vi "ErrHandler.vi"(1 "Err Code":u32=1, 2 "Action":enum16{"Init", "Process"}(ring)) -> (0 "Err Msg":string="OK!")   [LabVIEW 2011]
uses:
  Globals/CTCGlbs.vi
  Globals/DynaGlbs.vi
panel:
  in  "Incident #":i32=10
  in  "Lookup table":u32[](array[numeric])=[0, 1, 158, 159, 160, 165, 166, 167, 168, 169, 170, 178, 179, 180, 181, 182, 183, 184, 185, 186, 194, 195, 196, 205, 206, 215, 216, 235, 236, 246, 255]
  in  "Text messages":string="Failure\nOK!\nPort in use\nPort not found\nUnknown error\nIllegal stop bits\nIllegal word length\nIllegal parity setting\nIllegal baud rate\nWarning...\nSerial timeout\nNetwork in use\nBad network port\nEnd of file\nBad position\nBad object length\nBad object record\nFile not object\nFile wrong arch\nObject file not found\nRemote access error\nUnknown remote node\nUnsupported remote operation\nNot CT protocol\nBad response\nBad checksum\nOut of CT range\nNetwork not ready\nNetwork timeout\nWindows timer error\nUnknown network error"
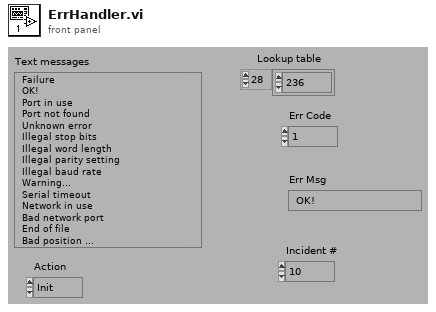
[diagram p1: front panel]
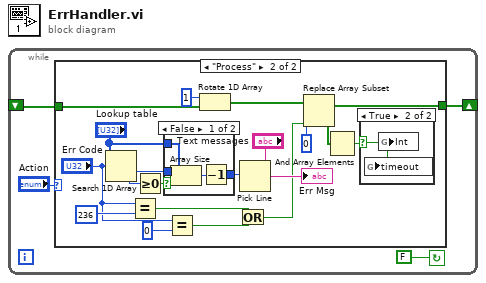
[diagram p0: block diagram]
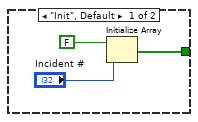
[diagram p2: hidden frame]
diagram:
  n1 = while {
    shift-left: _ -> [w2]
    shift-right: [w3] -> _
    stop <- FALSE continue-if-true
    n2 = case shown="\"Process\"" "Action" {
      tunnel: [w5 w18] -> w3
      tunnel: w2 -> [_ w20]
      frame "Init", Default {
        n3 = Initialize Array(FALSE, "Incident #") -> (w5:bool[])
      }
      frame "Process" {
        n4 = Search 1D Array(1D array="Lookup table", element="Err Code") -> (index of element=w24:i32)  [unwired: 1 in]
        n5 = Equal?(x="Err Code", y=u16 236) -> (x = y?=w10:bool)
        n6 = Greater Or Equal To 0?(x=w24) -> (x >= 0?=w25:bool)
        n7 = case shown="False" w25 {
          tunnel: w24 -> [_ w30]
          tunnel: [w27 w30] -> w13
          tunnel: "Lookup table" -> [w29 _]
          frame False {
            n8 = Array Size(array=w29) -> (size(s)=w28:i32)
            n9 = Decrement(x=w28) -> (x-1=w27:i32)
          }
          frame True {
          }
        }
        n10 = Equal?(x="Err Code", y=u16 0) -> (x = y?=w9:bool)
        n11 = Rotate 1D Array(1:w20, 2:i16 1) -> (0:w19:bool[])
        n12 = Or(x=w10, y=w9) -> (x .or. y?=w11:bool)
        n13 = Pick Line(multi-line string="Text messages", line index=w13) -> (output string=→"Err Msg":string)  [unwired: 1 in]
        n14 = Replace Array Subset(array=w19, new element=w11, index=0) -> (w18:bool[])
        n15 = And Array Elements(Boolean array=w18) -> (logical AND=w16:bool)
        n16 = case shown="True" w16 {
          selector: w16 -> [_ w26]
          frame False {
          }
          frame True {
            n17 = global write "CTCGlbs.vi" "timeout"(w26) -> ()
            n18 = global write "DynaGlbs.vi" "Int"(w26) -> ()
          }
        }
      }
    }
  }
